vi "show_&_clean_errors.vi"(8 "error in (no error)":errorcluster, 11 "message in":string) -> (0 "error out":errorcluster, 1 "Colors [4]":cluster{u32, u32}[](array[cluster]), 2 "status":bool, 3 "message out":string)   [LabVIEW 2015]
uses:
  <vilib>/Utility/error.llb/DialogType.ctl
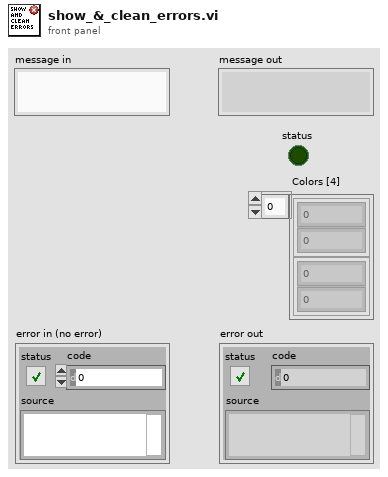
[diagram p1: front panel]
types:
  T1 = typedef "DialogType.ctl" = u16
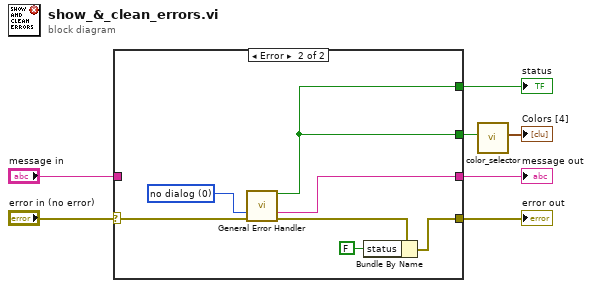
[diagram p0: block diagram]
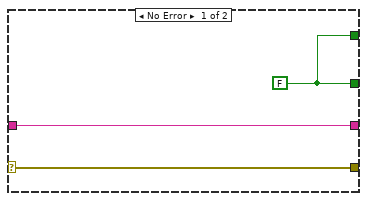
[diagram p2: hidden frame]
diagram:
  n1 = case shown="Error" "error in (no error)" {
    selector: "error in (no error)" -> [w10 w17]
    tunnel: [w9 w16] -> w2
    tunnel: [w10 w13] -> w3
    tunnel: "message in" -> [w9 _]
    tunnel: [w8 w11] -> w6
    tunnel: [w8 w11] -> w1
    frame No Error {
      w8 = FALSE
    }
    frame Error {
      w12 = T1 0 items=["no dialog", "OK message", "continue or stop message", "OK message + warnings", "continue/stop + warnings"] ("type of dialog (OK msg:1)")
      n2 = call <vilib>:"General Error Handler.vi"("type of dialog (OK msg:1)"=w12, "error in (no error)"=w17) -> ("error?"=w11:bool, "message"=w16:string, "error out"=w15:errorcluster)  [unwired: 9 in, 2 out]
      n3 = Bundle By Name(cluster=w15, "status"=FALSE) -> (w13:errorcluster)
    }
  }
  "error out" <- w3
  "message out" <- w2
  "status" <- w1
  n4 = call "color_selector.vi"("state"=w6) -> ("Colors [4]"=→"Colors [4]":cluster{u32, u32}[])  [unwired: 10 in]
